vi "GetDataType.vi"(8 "error in":errorcluster, 11 "Tunnel in":refnum<class "FlatSequenceInnerTunnel.lvclass">) -> (0 "error out":errorcluster, 2 "Data Type":variant, 3 "Tunnel out":refnum<class "FlatSequenceInnerTunnel.lvclass">)   [LabVIEW 2014, in "FlatSequenceInnerTunnel.lvclass"]
uses:
  FlatSequenceInnerTunnel.lvclass
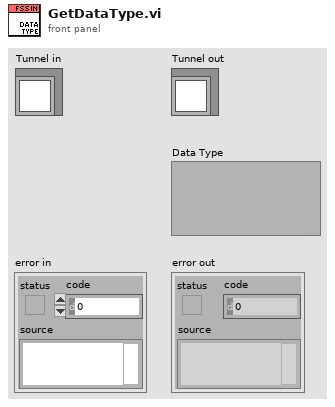
[diagram p1: front panel]
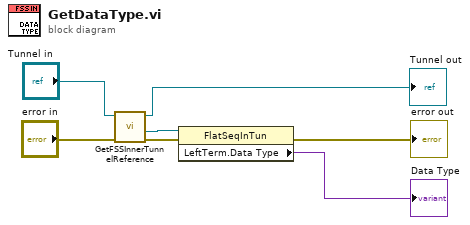
[diagram p0: block diagram]
diagram:
  n1 = call "GetFSSInnerTunnelReference.vi"("error in"="error in", "Tunnel in"="Tunnel in") -> ("error out"=w6:errorcluster, "reference out"=w7:refnum<vi>, "Tunnel out"=→"Tunnel out":refnum<class "FlatSequenceInnerTunnel.lvclass">)  [unwired: 7 in]
  n2 = property class="FlatSeqInTun"(reference=w7, error in=w6) -> (error out=→"error out":errorcluster, "LeftTerm.Data Type"=→"Data Type":variant)  [unwired: 1 out]
